vi "Image Size to Width DBL.vi"(11 "image size":T1) -> (3 "Numeric":dbl)   [LabVIEW 2015]
uses:
  <vilib>/Rock Robotics/WPI/Camera/WPI_CameraImageSize.ctl
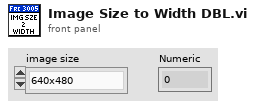
[diagram p1: front panel]
types:
  T1 = typedef "WPI_CameraImageSize.ctl" = enum16{"640x480", "320x240", "160x120", "Custom"}
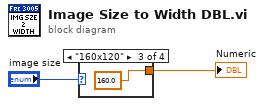
[diagram p0: block diagram]
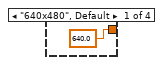
[diagram p2: hidden frame]
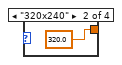
[diagram p3: hidden frame]
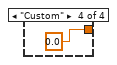
[diagram p4: hidden frame]
diagram:
  n1 = case shown="\"160x120\"" "image size" {
    tunnel: [640.0 320.0 160.0 0.0] -> w2
    frame "640x480", Default {
    }
    frame "320x240" {
    }
    frame "160x120" {
    }
    frame "Custom" {
    }
  }
  "Numeric" <- w2
